vi "IHL_Stop Collecting Helper.vi"() -> ()   [LabVIEW 2015, in "Tool Module.lvlib"]
uses:
  Tool Module.lvlib
  Tool Interface/Tool Interface.lvlib
panel:
  out "Success":bool
  out "CD Status":i32
  out "Array Size":u32
  out "error out":errorcluster
  in  "error in (no error)":errorcluster
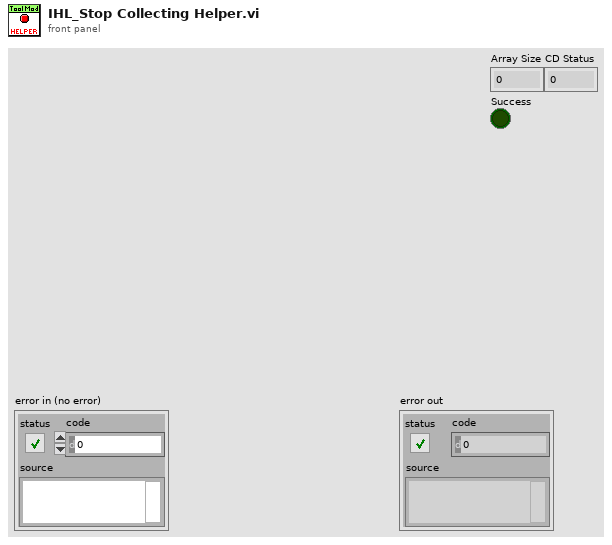
[diagram p1: front panel]
types:
  T1 = enum16{"Idle", "Receive HS Data", "Close Connection"}
  T2 = typedef "Tool Interface.lvlib/_Loop Ctrl Notifiers Cluster--typedef.ctl" = cluster{"Raw Stream Ctrl":refnum<notifier>}
  T3 = typedef "Tool Interface.lvlib/_HS Data Stream Params Cluster--typedef.ctl" = cluster{"Raw Data Stream Loop cmd":enum16{"Idle", "Receive HS Data", "Close Connection"}, "Data Array DVR ref":refnum<data-value>, "Sample Data notifier":refnum<notifier>, "Block Count Notifier":refnum<notifier>}
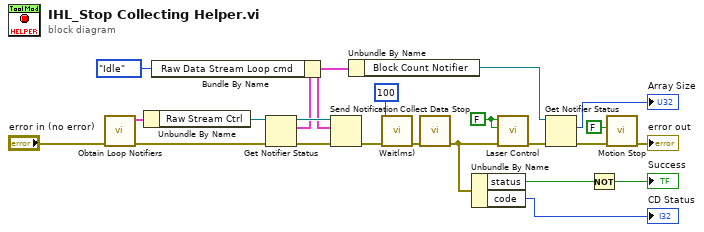
[diagram p0: block diagram]
diagram:
  w20 = FALSE ("Laser 1")
  n1 = call "Obtain Loop Notifiers.vi"("error in (no error)"="error in (no error)") -> ("error out"=w15:errorcluster, "Loop Ctrl Notifiers Cluster"=w17:T2)  [unwired: 9 in]
  n2 = Unbundle By Name(w17) -> ("Raw Stream Ctrl"=w16:refnum<notifier>)
  n3 = Get Notifier Status(notifier=w16, error in (no error)=w15) -> (notifier out=w13:refnum<notifier>, current notification=w11:T3, error out=w14:errorcluster)  [unwired: 2 out]
  n4 = Bundle By Name(cluster=w11, "Raw Data Stream Loop cmd"=T1."Idle" ("HS Data Stream SM enum")) -> (w9:T3)
  n5 = Send Notification(notification=w9, notifier=w13, error in (no error)=w14) -> (error out=w23:errorcluster)  [unwired: 1 out]
  n6 = Unbundle By Name(w9) -> ("Block Count Notifier"=w8:refnum<notifier>)
  n7 = call "Wait(ms).vi"("error in (no error)"=w23, "milliseconds"=u32 100) -> ("error out"=w22:errorcluster)  [unwired: 9 in]
  n8 = call "Collect Data Stop.vi"("error in (no error)"=w22) -> ("error out"=w7:errorcluster)  [unwired: 10 in]
  n9 = Unbundle By Name(w7) -> ("status"=w2:bool, "code"=→"CD Status":i32)
  n10 = call "Laser Control.vi"("error in (no error)"=w7, "Laser 2"=w20, "Laser 1"=w20) -> ("error out"=w18:errorcluster)  [unwired: 8 in]
  n11 = Get Notifier Status(notifier=w8, error in (no error)=w18) -> (current notification=→"Array Size":u32, error out=w21:errorcluster)  [unwired: 3 out]
  n12 = Not(x=w2) -> (.not. x?=→"Success":bool)
  n13 = call "Motion Stop.vi"("error in (no error)"=w21, "Decel?"=FALSE) -> ("error out"=→"error out":errorcluster)  [unwired: 9 in]
